vi "destroy.vi"(8 "error in (no error)":errorcluster, 11 "XY Stage Class in":refnum<class "XY Stage Class.lvclass">) -> (0 "error out":errorcluster, 3 "XY Stage Class out":refnum<class "XY Stage Class.lvclass">)   [LabVIEW 2022 SP3, in "XY Stage Class.lvclass"]
uses:
  XY Stage Class.lvclass
  XY Stage Class.lvclass/XY Stage Class.ctl
  iView/base view/base view.lvclass
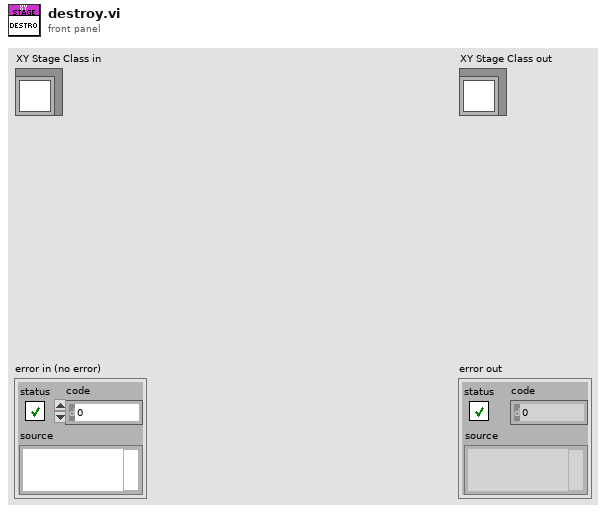
[diagram p1: front panel]
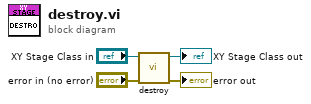
[diagram p0: block diagram]
diagram:
  n1 = call-parent "destroy.vi"("error in (no error)"="error in (no error)", "base view in"="XY Stage Class in") -> ("error out"=→"error out":errorcluster, "base view out"=→"XY Stage Class out":refnum<class "XY Stage Class.lvclass">)  [unwired: 8 in]
